vi "Write Control Systems.vi"(8 "error in (no error)":errorcluster, 10 "Control Systems":T1(array[cluster]), 11 "Manager in":refnum<class "Manager.lvclass">) -> (0 "error out":errorcluster, 3 "Manager out":refnum<class "Manager.lvclass">)   [LabVIEW 2013, in "Manager.lvlib" / "Manager.lvclass"]
uses:
  Manager.lvclass
  PluginInterface/Actor Framework.lvlibp/Message Enqueuer/Message Enqueuer.lvclass
  Manager.lvclass/Manager.ctl
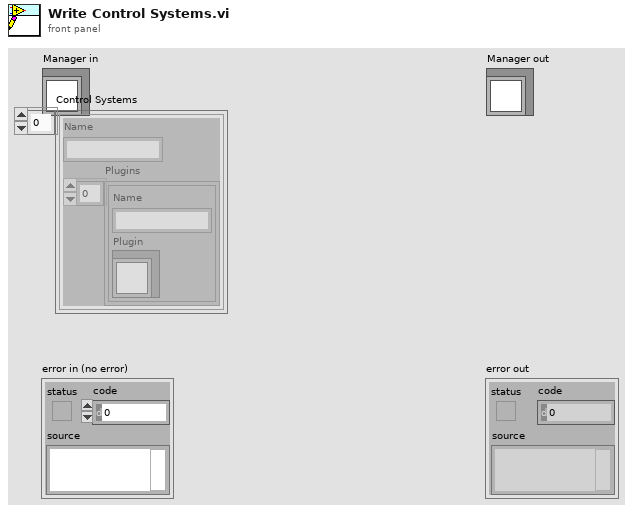
[diagram p1: front panel]
types:
  T1 = cluster{"Name":string, "Plugins":cluster{"Name":string, "Plugin":refnum<class "Message Enqueuer.lvclass">}[]}[]
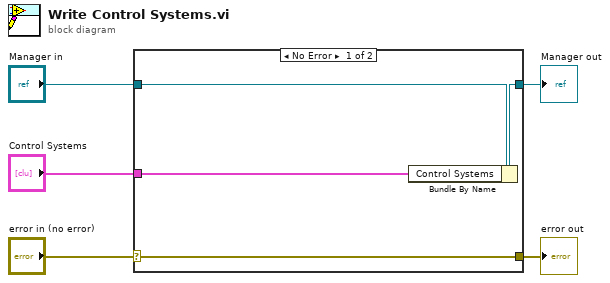
[diagram p0: block diagram]
diagram:
  n1 = case shown="No Error" "error in (no error)" {
    selector: "error in (no error)" -> [w9 w10]
    tunnel: [w9 w10] -> w4
    tunnel: [w7 w11] -> w2
    tunnel: "Manager in" -> [w8 w11]
    tunnel: "Control Systems" -> [w6 _]
    frame No Error {
      n2 = Bundle By Name(cluster=w8, "Control Systems"=w6) -> (w7:refnum<class "Manager.lvclass">)
    }
    frame Error {
    }
  }
  "error out" <- w4
  "Manager out" <- w2
